vi "Sharing_client_status.vi"(2 "Ch Names":string[](array[string]), 3 "Values":dbl[](array[numeric]) format="%.2f", 4 "Client Name":string) -> (0 "Active Machines in Rig":bool, 1 "Active Machines in Group":bool)   [LabVIEW 2010]
uses:
  ADAM_Global.vi
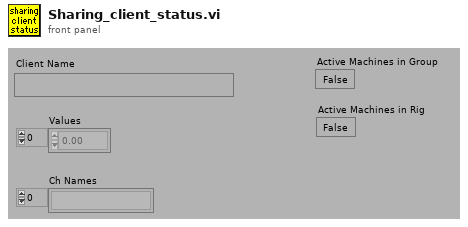
[diagram p1: front panel]
types:
  T1 = typedef "Client_State_Cluster.ctl" = cluster{"Client Name":string, "Traverse level State":T2, "People to Email":string[], "Next Contact Time":dbl}
  T2 = typedef "Traverse_Level_State.ctl" = enum16{"Running", "Complete"}
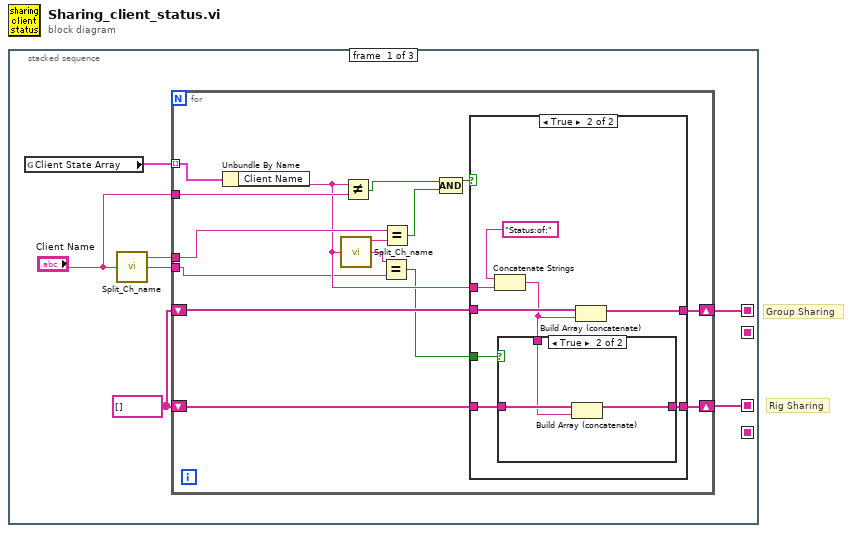
[diagram p0: block diagram]
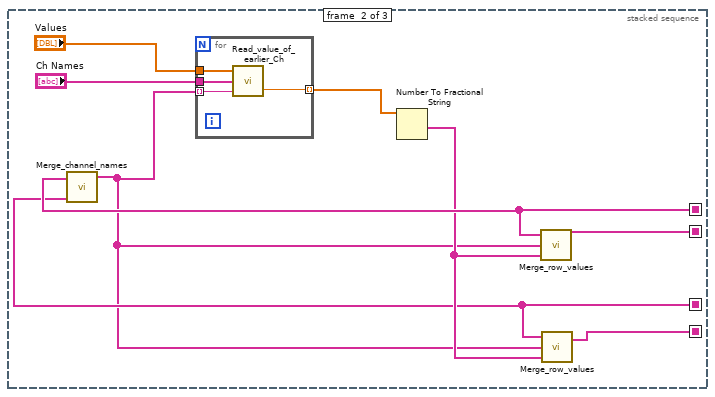
[diagram p4: hidden frame]
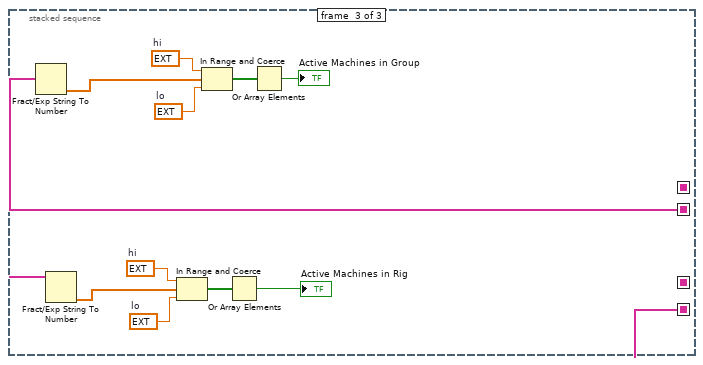
[diagram p5: hidden frame]
diagram:
  # "Rig Sharing"
  # "Group Sharing"
  n1 = stacked-sequence {
    seq-local: [w2 _ _] -> [_ w45 _]
    seq-local: [w1 _ _] -> [_ w42 _]
    seq-local: [_ w44 _] -> [_ _ w59]
    seq-local: [_ w41 _] -> [_ _ w51]
    frame #0 {
      w3 = string[] []
      n2 = global read "ADAM_Global.vi" "Client State Array"() -> (w7:T1[])
      n3 = call "Split_Ch_name.vi"("Ch name"="Client Name") -> ("Top level"=w5:string, "Middle"=w4:string)  [unwired: 1 out]
      n4 = for {
        tunnel: w7 -> [w22] mode=indexing
        tunnel: "Client Name" -> [w21]
        tunnel: w5 -> [w19]
        shift-right: [w13] -> w2
        shift-left: w3 -> [w15]
        tunnel: w4 -> [w11]
        shift-right: [w8] -> w1
        shift-left: w3 -> [w9]
        n5 = Unbundle By Name(w22) -> ("Client Name"=w14:string)
        n6 = call "Split_Ch_name.vi"("Ch name"=w14) -> ("Top level"=w20:string, "Middle"=w12:string)  [unwired: 1 out]
        n7 = Not Equal?(x=w14, y=w21) -> (x != y?=w17:bool)
        n8 = Equal?(x=w12, y=w11) -> (x = y?=w10:bool)
        n9 = Equal?(x=w19, y=w20) -> (x = y?=w18:bool)
        n10 = Compound Arithmetic op=AND(w17, w18) -> (w16:bool)
        n11 = case shown="True" w16 {
          tunnel: w15 -> [w24 w32]
          tunnel: w14 -> [_ w27]
          tunnel: [w24 w31] -> w13
          tunnel: w10 -> [_ w30]
          tunnel: w9 -> [w23 w29]
          tunnel: [w23 w28] -> w8
          frame False {
          }
          frame True {
            n12 = Concatenate Strings("Status:of:" ("Substring"), w27) -> (w26:string)
            n13 = case shown="True" w30 {
              tunnel: w29 -> [w33 w36]
              tunnel: [w33 w35] -> w28
              tunnel: w26 -> [_ w34]
              frame False {
              }
              frame True {
                n14 = Build Array (concatenate)(w36, w34) -> (w35:string[])
              }
            }
            n15 = Build Array (concatenate)(w32, w26) -> (w31:string[])
          }
        }
      }
    }
    frame #1 {
      n16 = call "Merge_channel_names.vi"("Preferred Channel array"=w45, "Channel array"=w42) -> ("Merged Channels"=w38:string[])  [unwired: 2 out]
      n17 = for {
        tunnel: "Values" -> [w49]
        tunnel: "Ch Names" -> [w48]
        tunnel: w38 -> [w47] mode=indexing
        tunnel: [w46] -> w37 mode=indexing
        n18 = call "Read_value_of_earlier_Ch.vi"("Desired Ch to Read"=w47, "Ch names"=w48, "Present scan array"=w49) -> ("Value"=w46:dbl)  [unwired: 1 in, 1 out]
      }
      n19 = Number To Fractional String(number=w37) -> (F-format string=w43:string[])  [unwired: 3 out]
      n20 = call "Merge_row_values.vi"("Present Row values"=w43, "Present Channels"=w38, "Desired Channels"=w45) -> ("Desired Row values"=w44:string[])  [unwired: 1 out]
      n21 = call "Merge_row_values.vi"("Present Row values"=w43, "Present Channels"=w38, "Desired Channels"=w42) -> ("Desired Row values"=w41:string[])  [unwired: 1 out]
    }
    frame #2 {
      w53 = ext 5.5  # hi
      w54 = ext 2.5  # lo
      w60 = ext 2.5  # lo
      w61 = ext 5.5  # hi
      n22 = Fract/Exp String To Number(string=w59) -> (number=w58:dbl[])  [unwired: 4 out]
      n23 = Fract/Exp String To Number(string=w51) -> (number=w52:dbl[])  [unwired: 4 out]
      n24 = In Range and Coerce(upper limit=w53, x=w52, lower limit=w54) -> (In Range?=w55:bool[])  [unwired: 1 out]
      n25 = In Range and Coerce(upper limit=w61, x=w58, lower limit=w60) -> (In Range?=w57:bool[])  [unwired: 1 out]
      n26 = Or Array Elements(Boolean array=w55) -> (logical OR=→"Active Machines in Rig":bool)
      n27 = Or Array Elements(Boolean array=w57) -> (logical OR=→"Active Machines in Group":bool)
    }
  }
